vi "HexapodCloseHardware.vi"(8 "error in (no error)":errorcluster, 11 "C-887 in":refnum<class "C-887.lvclass">) -> (0 "error out":errorcluster)   [LabVIEW 2020, in "C-887.lvclass"]
uses:
  C-887.lvclass
  C-887.lvclass/C-887.ctl
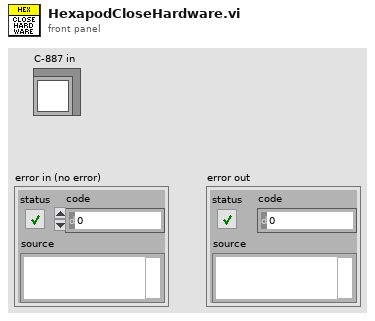
[diagram p1: front panel]
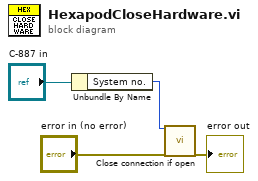
[diagram p0: block diagram]
diagram:
  n1 = Unbundle By Name("C-887 in") -> ("System no."=w1:i32)
  n2 = call "Close connection if open.vi"("System no."=w1, "error in"="error in (no error)") -> ("error out"=→"error out":errorcluster)  [unwired: 1 in, 16 out]
